vi "gRPC_ATS.vi"(11 "CommandLineIn":string[](array[string])) -> (2 "source":string, 3 "return code":i32)   [LabVIEW 2019]
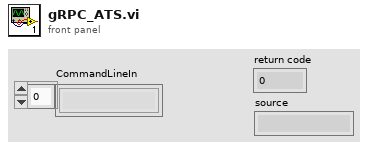
[diagram p1: front panel]
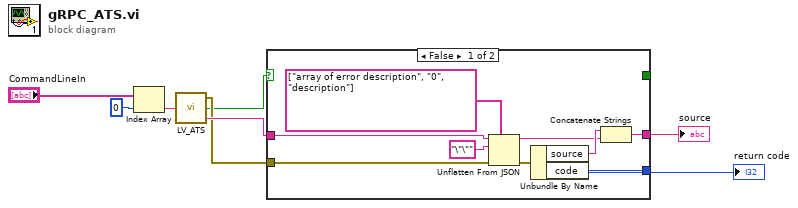
[diagram p0: block diagram]
diagram:
  n1 = Index Array(array="CommandLineIn", index=0) -> (element=w7:string)
  n2 = call "LV_ATS.vi"("test json in"=w7) -> ("formatted test json out"=w3:string, "PASS"=w1:bool, "error out"=w2:errorcluster)  [unwired: 1 in, 1 out]
  n3 = case shown="False" w1 {
    selector: w1 -> [_ w18]
    tunnel: [_ w18] -> _
    tunnel: w3 -> [w17 _]
    tunnel: w2 -> [w11 _]
    tunnel: [w9 _] -> w4
    tunnel: [w15 _] -> w5
    frame False {
      n4 = Unflatten From JSON(path=string[] ["array of error description", "0", "description"], JSON string=w17, type and defaults="\"\"", error in (no error)=w11) -> (value=w13:string, error out=w10:errorcluster)  [unwired: 3 in]
      n5 = Unbundle By Name(w10) -> ("source"=w16:string, "code"=w15:i32)
      n6 = Concatenate Strings(w16, w13) -> (w9:string)
    }
    frame True {
    }
  }
  "return code" <- w5
  "source" <- w4
